vi "Read OUR calculation threshold.vi"(8 "error in (no error)":errorcluster, 11 "OUR_Monitor in":refnum<class "OUR_Monitor.lvclass">) -> (0 "error out":errorcluster, 2 "OUR calculation threshold":dbl, 3 "OUR_Monitor out":refnum<class "OUR_Monitor.lvclass">)   [LabVIEW 2021, in "MBPOnOff_Controller.lvlib" / "OUR_Monitor.lvclass"]
uses:
  OUR_Monitor.lvclass
  OUR_Monitor.lvclass/OUR_Monitor.ctl
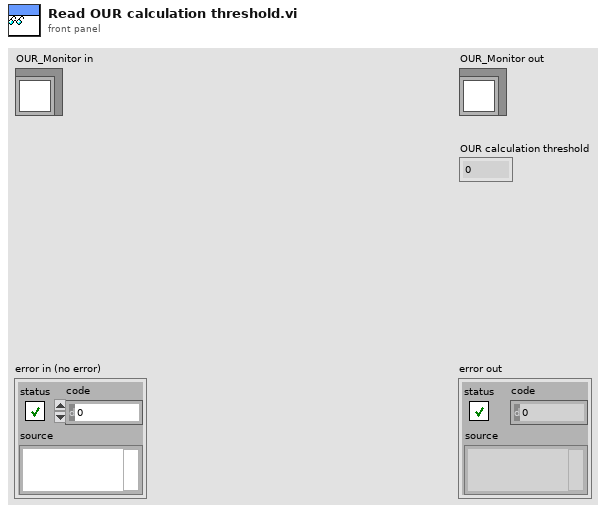
[diagram p1: front panel]
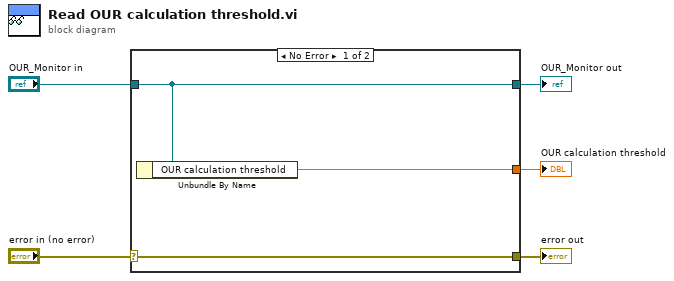
[diagram p0: block diagram]
diagram:
  n1 = case shown="No Error" "error in (no error)" {
    selector: "error in (no error)" -> [w8 w9]
    tunnel: [w8 w9] -> w4
    tunnel: [w7 w10] -> w2
    tunnel: "OUR_Monitor in" -> [w7 w10]
    tunnel: [w6 _] -> w1
    frame No Error {
      n2 = Unbundle By Name(w7) -> ("OUR calculation threshold"=w6:dbl)
    }
    frame Error {
    }
  }
  "error out" <- w4
  "OUR_Monitor out" <- w2
  "OUR calculation threshold" <- w1
